vi "2 OverrideSetpoints.vi"() -> (2 "Setpoints Out":T1)   [LabVIEW 2011]
doc: "The OverrideSetpoints VI simply unpacks the Manual Override Cluster global as sent by the OCU. The outputs of the VI are the manual setpoints and whether or not the think loop should consider them."
uses:
  2 Typedefs/setpoints to boat.ctl
  2 Typedefs/sail setpt.ctl
  2 Typedefs/rudder angle.ctl
  2 Typedefs/setpoints to arbiter.ctl
  2 Globals/2 Global.vi
panel:
  out "Override Active Rudder":bool
  out "Override Active Sail":bool
  out "Override Setpoints":T2
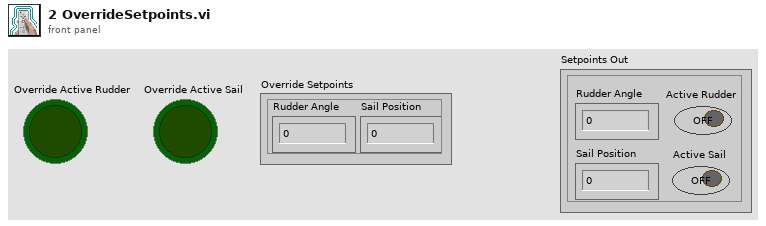
[diagram p1: front panel]
types:
  T1 = typedef "setpoints to arbiter.ctl" = cluster{"Rudder Angle":dbl, "Sail Position":dbl, "Active Rudder":bool, "Active Sail":bool}
  T2 = typedef "setpoints to boat.ctl" = cluster{"Sail Position":T3, "Rudder Angle":T4}
  T3 = typedef "sail setpt.ctl" = dbl
  T4 = typedef "rudder angle.ctl" = dbl
  T5 = typedef "manual override.ctl" = cluster{"Override Active Rudder":bool, "Setpoints":T2, "Override Active Sail":bool}
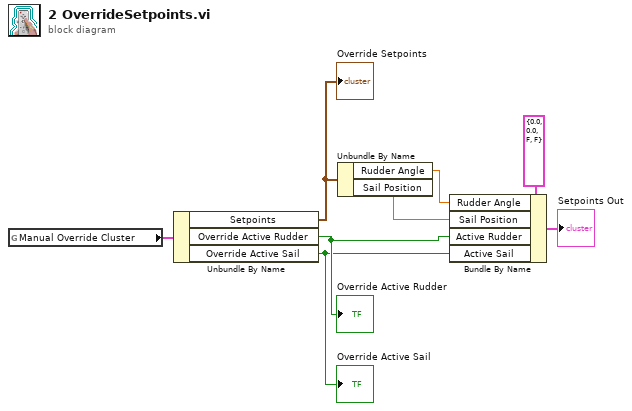
[diagram p0: block diagram]
diagram:
  n1 = global read "2 Global.vi" "Manual Override Cluster"() -> (w8:T5)
  n2 = Unbundle By Name(w8) -> ("Setpoints"=w3:T2, "Override Active Rudder"=w7:bool, "Override Active Sail"=w4:bool)
  "Override Setpoints" <- w3
  "Override Active Sail" <- w4
  "Override Active Rudder" <- w7
  n3 = Unbundle By Name(w3) -> ("Rudder Angle"=w2:T4, "Sail Position"=w1:T3)
  n4 = Bundle By Name(cluster=T1 {"Rudder Angle"=0.0, "Sail Position"=0.0, "Active Rudder"=FALSE, "Active Sail"=FALSE} ("Setpoints Out"), "Rudder Angle"=w2, "Sail Position"=w1, "Active Rudder"=w7, "Active Sail"=w4) -> (→"Setpoints Out":T1)
